vi "display_and_capture_pattern.vi"(5 "flip direction":bool, 7 "capture images ?":bool=TRUE, 9 "intial phase shift":dbl, 10 "#fringes":dbl=5.0, 11 "#Phase Shifts":i32=4) -> (1 "ul_ar_pxar_capt_images":u8[][][](array[numeric]), 2 "ul_ar_pxar_orig_pattern":u8[][][](array[numeric]))   [LabVIEW 2011]
doc: "This VIs displays the fringe pattern on the screen and records images of that pattern. Those images are converted to arrays and transpose for the horizontal fringes (for simplified handling later)"
uses:
  <vilib>/vision/Image Controls.llb/IMAQ Image.ctl
  global_vars.vi
  <vilib>/vision/NI_Vision_Development_Module.lvlib
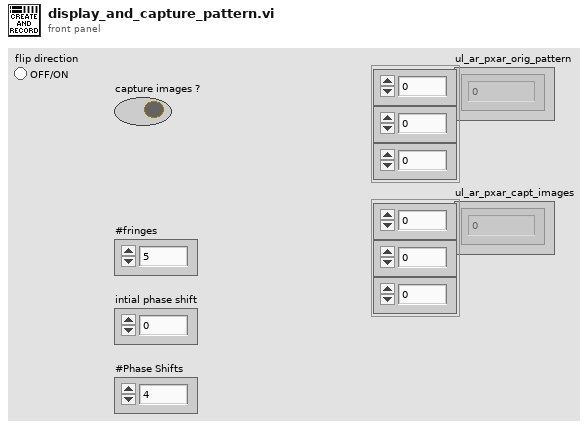
[diagram p1: front panel]
types:
  T1 = typedef "IMAQ Image.ctl" = refnum<image>
  T2 = cluster{"radius correction":i16, "u8_x_center_cor":i16, "u8_y_center_cor":i16}
  T3 = typedef "Image Type" = u32
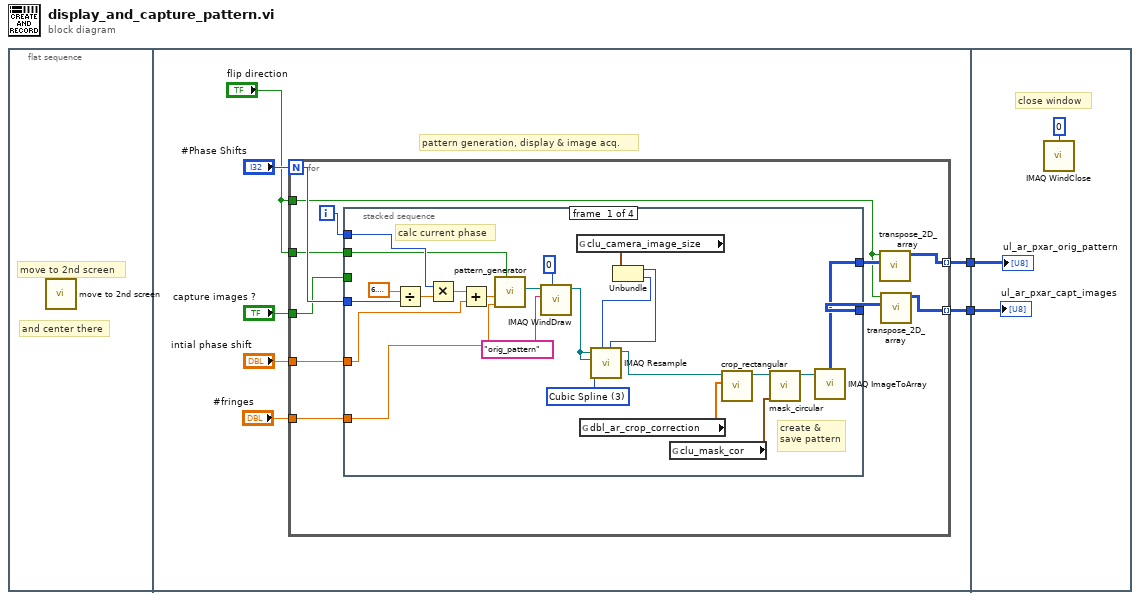
[diagram p0: block diagram]
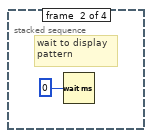
[diagram p2: hidden frame]
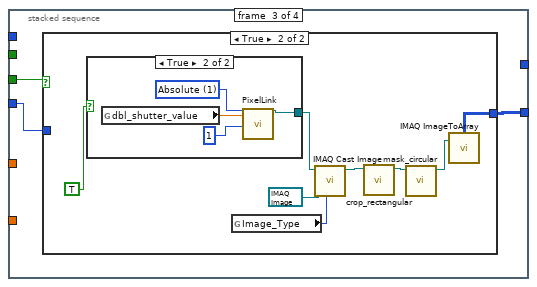
[diagram p3: hidden frame]
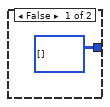
[diagram p4: hidden frame]
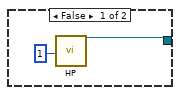
[diagram p5: hidden frame]
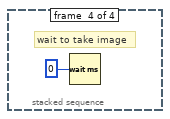
[diagram p6: hidden frame]
diagram:
  n1 = flat-sequence {
    tunnel: [w5] -> w2
    tunnel: [w4] -> w1
    tunnel: w2 -> [w65]
    tunnel: w1 -> [w66]
    frame #0 {
      # "and center there"
      # "move to 2nd screen"
      n2 = call "move to 2nd screen.vi"() -> ()  [unwired: 12 in]
    }
    frame #1 {
      # "pattern generation, display & image acq."
      n3 = for {
        N: "#Phase Shifts" -> [w20]
        tunnel: [w13] -> w4 mode=indexing
        tunnel: [w11] -> w5 mode=indexing
        tunnel: "#fringes" -> [w18]
        tunnel: "intial phase shift" -> [w17]
        tunnel: "capture images ?" -> [w16]
        tunnel: "flip direction" -> [w15]
        tunnel: "flip direction" -> [w10]
        i -> [w19]
        n4 = stacked-sequence {
          tunnel: w20 -> [w35 _ w46 _]
          tunnel: [w40 _ _ _] -> w14
          tunnel: [_ _ w45 _] -> w12
          tunnel: w19 -> [w36 _ _ _]
          tunnel: w18 -> [w33 _ _ _]
          tunnel: w17 -> [w32 _ _ _]
          tunnel: w16 -> [_ _ w47 _]
          tunnel: w15 -> [w31 _ _ _]
          frame #0 {
            w24 = u32 3 items=["Zero Order", "Bi-Linear", "Quadratic", "Cubic Spline"] ("Interpolation Type")
            # "calc current phase"
            # "create & \nsave pattern"
            n5 = Divide(x=6.283185307179586, y=w35) -> (x/y=w38:dbl)
            n6 = Multiply(x=w36, y=w38) -> (x*y=w37:dbl)
            n7 = Add(x=w37, y=w32) -> (x+y=w34:dbl)
            n8 = call "pattern_generator.vi"("flip direction"=w31, "fringe number"=w33, "phase"=w34) -> ("fringe pattern"=w41:T1)  [unwired: 7 in, 1 out]
            n9 = call "IMAQ WindDraw"("Window Number (0...15)"=0, "Title"="orig_pattern", "Image"=w41) -> ("Image Out (duplicate)"=w25:T1)  [unwired: 7 in, 1 out]
            n10 = global read "global_vars.vi" "clu_camera_image_size"() -> (w23:cluster{"Width":u32, "Height":u32})
            n11 = global read "global_vars.vi" "dbl_ar_crop_correction"() -> (w28:dbl[])
            n12 = Unbundle(w23) -> ("Width"=w22:u32, "Height"=w21:u32)
            n13 = call "IMAQ Resample"("X Resolution"=w22, "Y Resolution"=w21, "Interpolation Type"=w24, "Image Dst"=w25, "Image Src"=w25) -> ("Image Dst Out"=w26:T1)  [unwired: 5 in, 1 out]
            n14 = global read "global_vars.vi" "clu_mask_cor"() -> (w27:T2)
            n15 = call "crop_rectangular.vi"("dbl_ar_crop_correction"=w28, "image_in"=w26) -> ("cropped image out"=w30:T1)  [unwired: 8 in, 1 out]
            n16 = call "mask_circular.vi"("clu_mask_cor"=w27, "image in"=w30) -> ("masekd image out"=w29:T1)  [unwired: 9 in]
            n17 = call "IMAQ ImageToArray"("Image"=w29) -> ("Image Pixels (U8)"=w40:u8[][])  [unwired: 3 in, 4 out]
          }
          frame #1 {
            # "wait to display \npattern"
            n18 = Wait (ms)(milliseconds to wait=u32 0) -> ()  [unwired: 1 out]
          }
          frame #2 {
            n19 = case shown="True" w47 {
              tunnel: w46 -> [_ _]
              tunnel: [u8[][] [] ("Image Pixels (U8)") w50] -> w45
              frame False {
              }
              frame True {
                n20 = case shown="True" TRUE {
                  tunnel: [w57 w59] -> w54
                  frame False {
                    n21 = call "HP"("Number of Images"=1) -> ("Image Out"=w57:T1)  [unwired: 24 in, 2 out]
                  }
                  frame True {
                    w61 = u32 1 items=["Absolute"=1, "Auto"=3, "Relative"=0, "One Push"=4, "Ignored"=5] ("Shutter::Mode")
                    n22 = global read "global_vars.vi" "dbl_shutter_value"() -> (w60:dbl)
                    n23 = call "PixelLink"("Shutter::Mode"=w61, "Shutter::Value"=w60, "Number of Images"=1) -> ("Image Out"=w59:T1)  [unwired: 22 in, 2 out]
                  }
                }
                n24 = global read "global_vars.vi" "Image_Type"() -> (w56:T3)
                n25 = call "IMAQ Cast Image"("Image Type"=w56, "Image Dst"=T1 refnum, "Image Src"=w54) -> ("Image Dst Out"=w53:T1)  [unwired: 7 in, 1 out]
                n26 = call "crop_rectangular.vi"("image_in"=w53) -> ("cropped image out"=w52:T1)  [unwired: 9 in, 1 out]
                n27 = call "mask_circular.vi"("image in"=w52) -> ("masekd image out"=w51:T1)  [unwired: 10 in]
                n28 = call "IMAQ ImageToArray"("Image"=w51) -> ("Image Pixels (U8)"=w50:u8[][])  [unwired: 3 in, 4 out]
              }
            }
          }
          frame #3 {
            # "wait to take image"
            n29 = Wait (ms)(milliseconds to wait=u32 0) -> ()  [unwired: 1 out]
          }
        }
        n30 = call "transpose_2D_array.vi"("Image Pixels (U8) in"=w14, "flip direction"=w10) -> ("Image Pixels (U8) out"=w13:u8[][])  [unwired: 9 in]
        n31 = call "transpose_2D_array.vi"("Image Pixels (U8) in"=w12, "flip direction"=w10) -> ("Image Pixels (U8) out"=w11:u8[][])  [unwired: 9 in]
      }
    }
    frame #2 {
      # "close window"
      n32 = call "IMAQ WindClose"("Window Number (0...15)"=0) -> ()  [unwired: 5 in, 1 out]
      "ul_ar_pxar_orig_pattern" <- w66
      "ul_ar_pxar_capt_images" <- w65
    }
  }
